vi "chainManyCommands.vi"(9 "Comments":string, 10 "CommandArray":T1, 11 "String in in":string) -> (3 "String out":string)   [LabVIEW 2013]
uses:
  commandArray.ctl
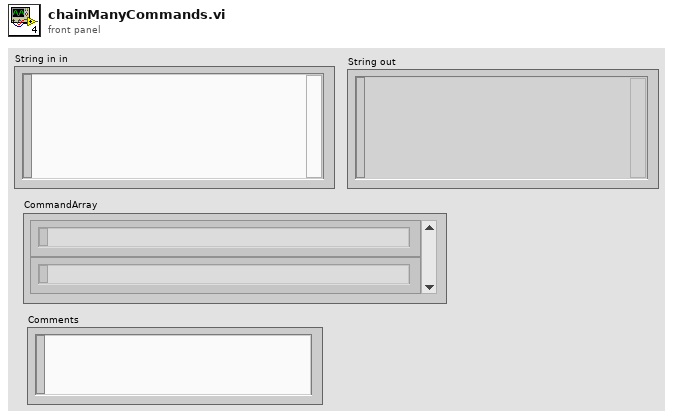
[diagram p1: front panel]
types:
  T1 = typedef "commandArray.ctl" = string[]
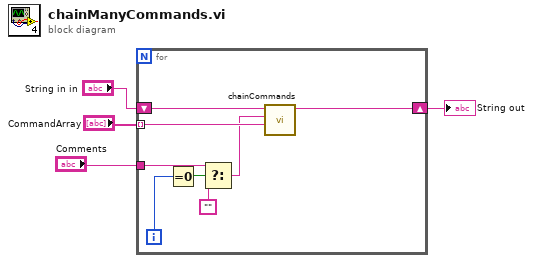
[diagram p0: block diagram]
diagram:
  n1 = for {
    shift-right: [w12] -> w4
    shift-left: "String in in" -> [w11]
    tunnel: "CommandArray" -> [w10] mode=indexing
    tunnel: "Comments" -> [w7]
    i -> [w9]
    n2 = Equal To 0?(x=w9) -> (x = 0?=w8:bool)
    n3 = Select(t=w7, s=w8, f="") -> (s? t:f=w5:string)
    n4 = call "chainCommands.vi"("Command"=w10, "Comments"=w5, "StringIn"=w11) -> ("StringOut"=w12:string)  [unwired: 8 in]
  }
  "String out" <- w4
